vi "Create Test Method Dialog.vi"(11 "Class Ref":refnum<vi>) -> ()   [LabVIEW 2013, in "Scripter.lvlib"]
uses:
  Scripter.lvlib
  _td Dialog Data.ctl
panel:
  out "Methods List":string[](array[string])
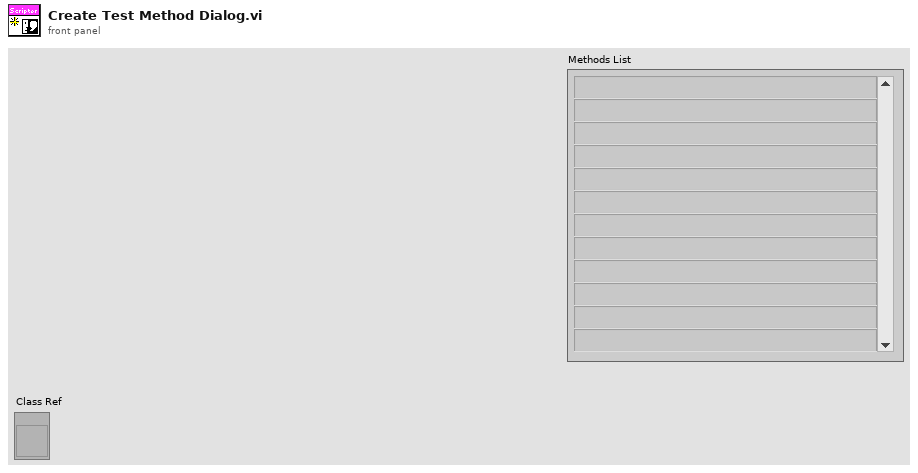
[diagram p1: front panel]
types:
  T1 = enum32{"Invalid", "Standard", "Closed", "Hidden", "Minimized", "Maximized"}
  T2 = enum32{"invalid app kind", "Development System", "Run Time System", "Student Edition", "Embedded LabVIEW", "Evaluation", "Custom"}
  T3 = typedef "Scripter.lvlib/_td Dialog Data.ctl" = cluster{"Core":cluster{"Current VI Reference":refnum<vi>, "Close Panel on Exit?":bool}, "Class Ref":refnum<vi>, "Class Folder Path":path, "Method Name":string, "Methods List":string[], "Templates Folder Path":path, "Template VIs":path[], "Template VIs List":string[], "Use Template?":bool}
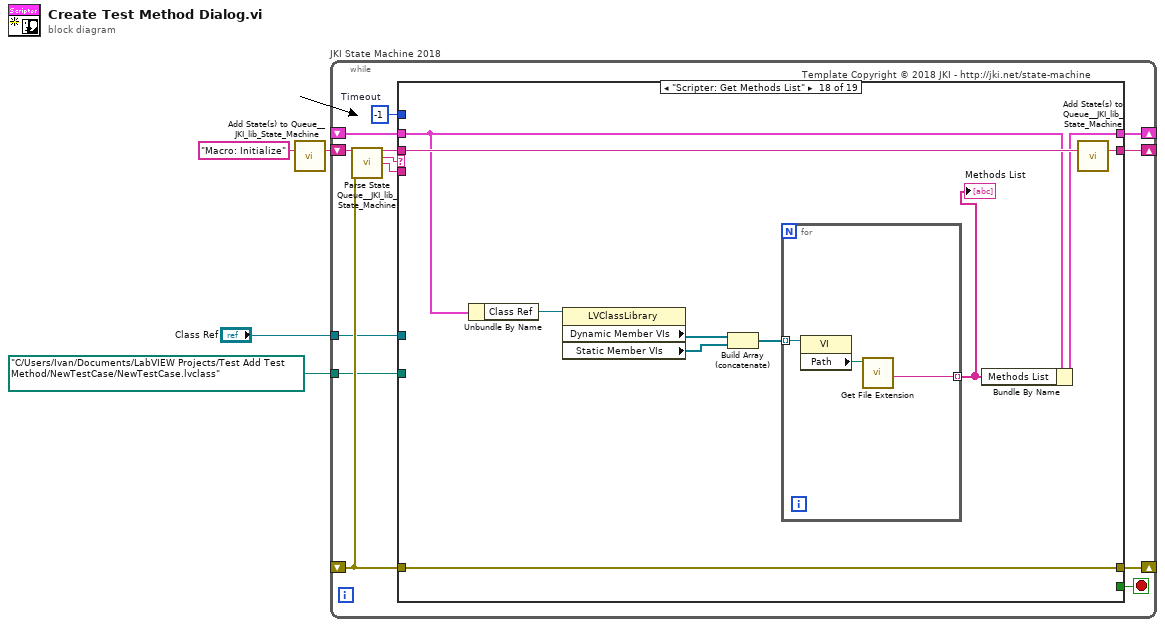
[diagram p0: block diagram]
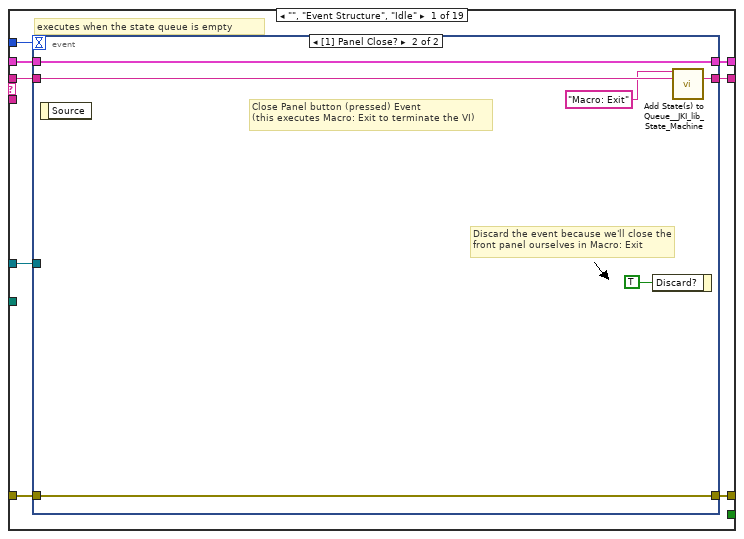
[diagram p2: hidden frame]
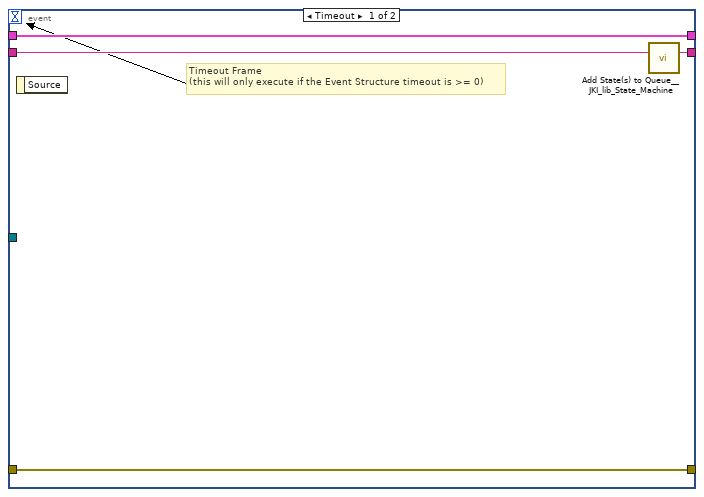
[diagram p3: hidden frame]
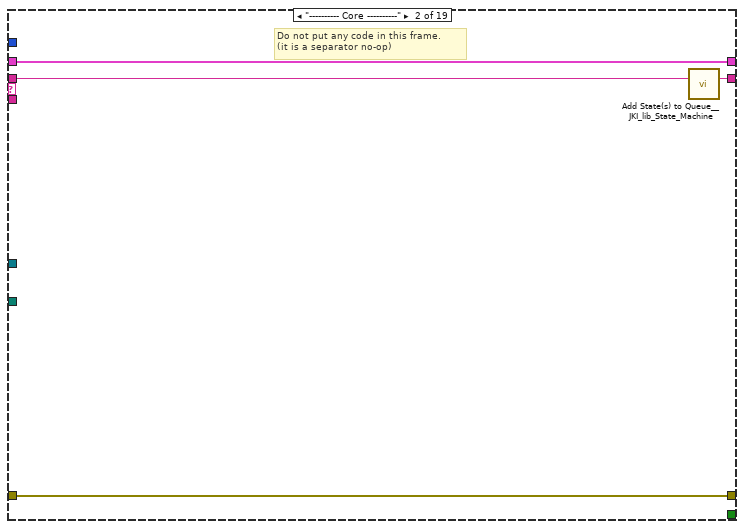
[diagram p4: hidden frame]
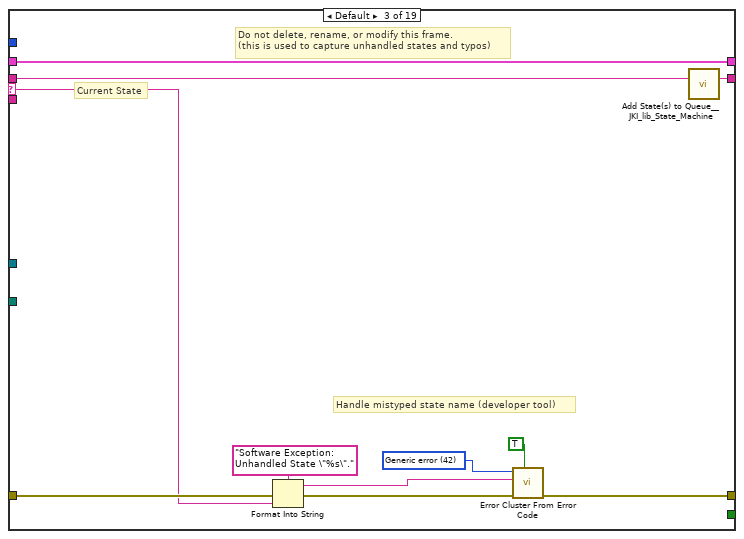
[diagram p5: hidden frame]
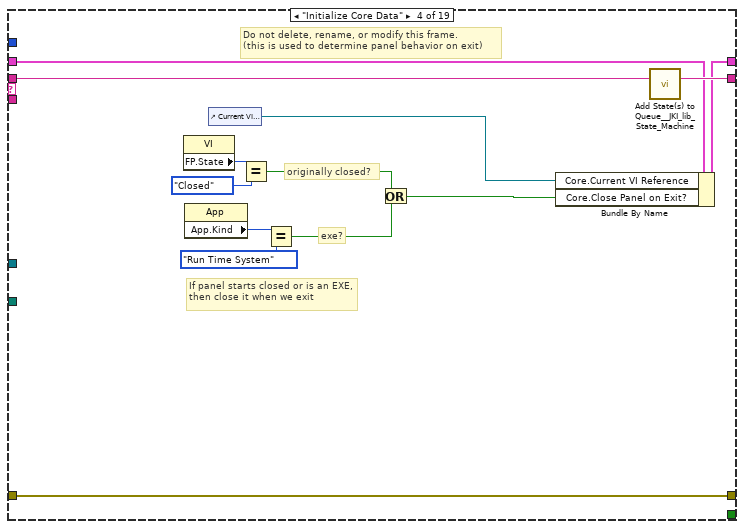
[diagram p6: hidden frame]
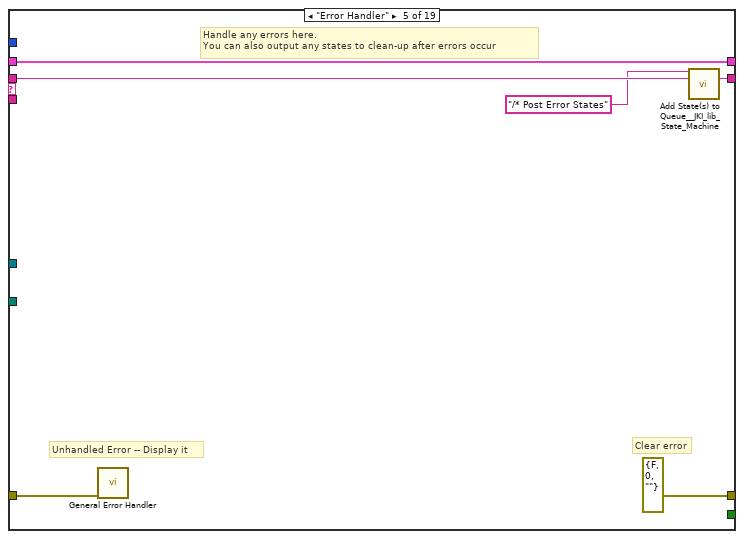
[diagram p7: hidden frame]
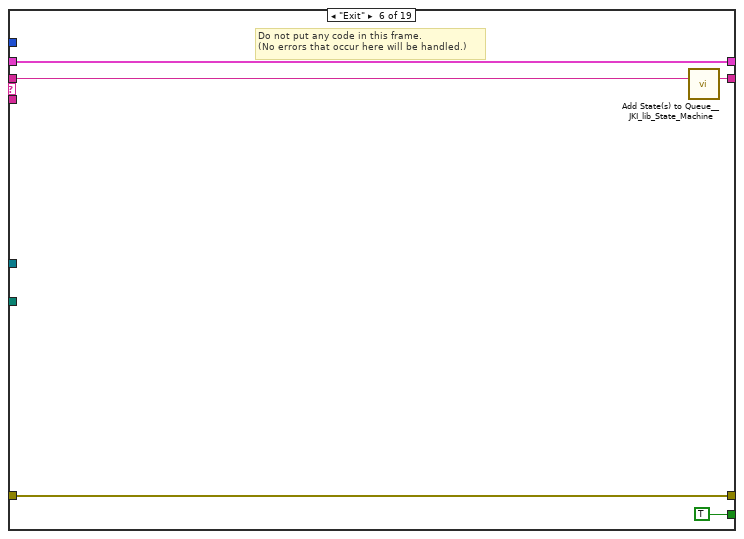
[diagram p8: hidden frame]
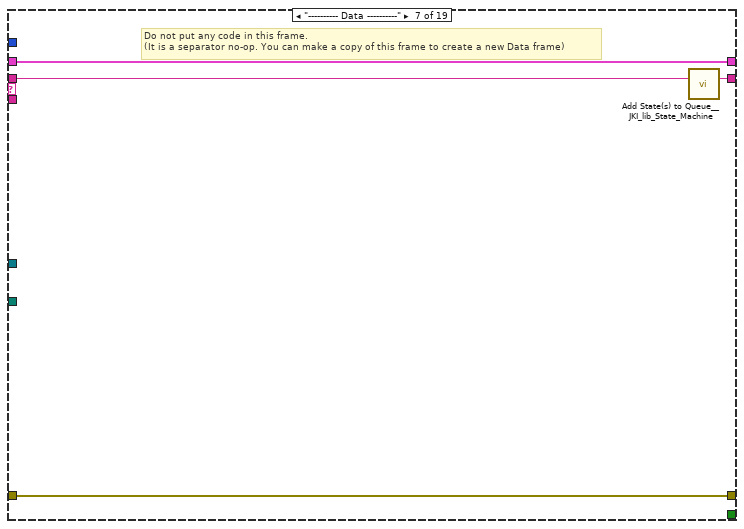
[diagram p9: hidden frame]
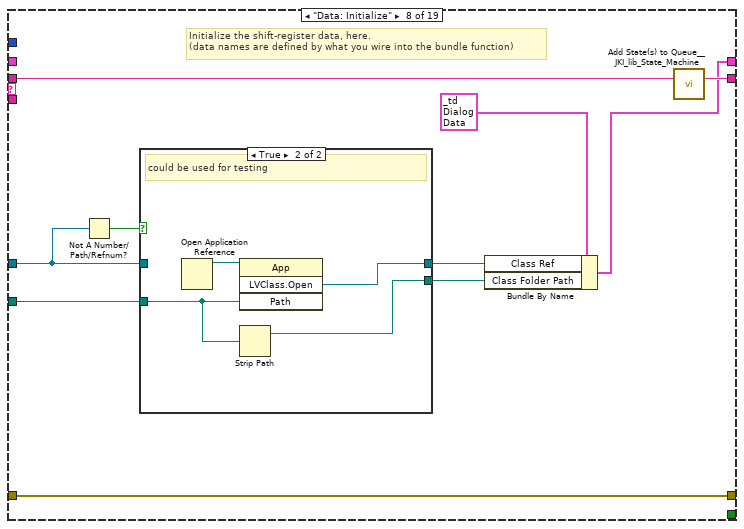
[diagram p10: hidden frame]
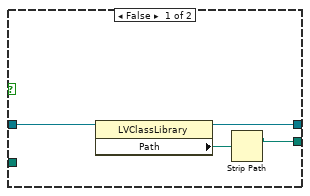
[diagram p11: hidden frame]
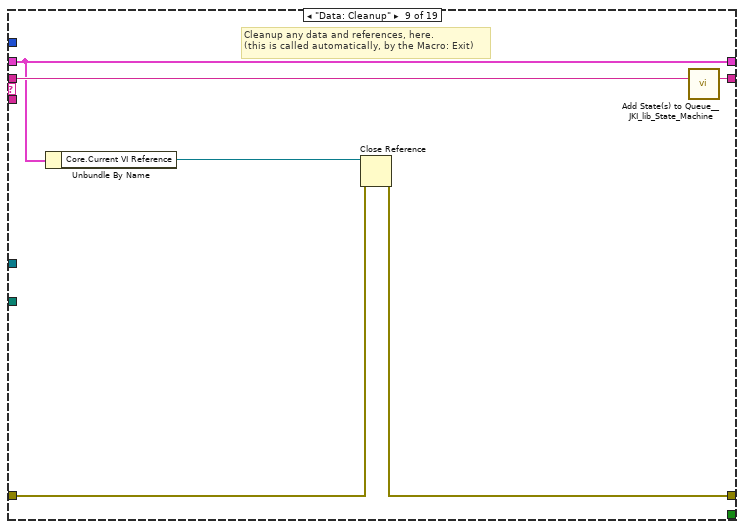
[diagram p12: hidden frame]
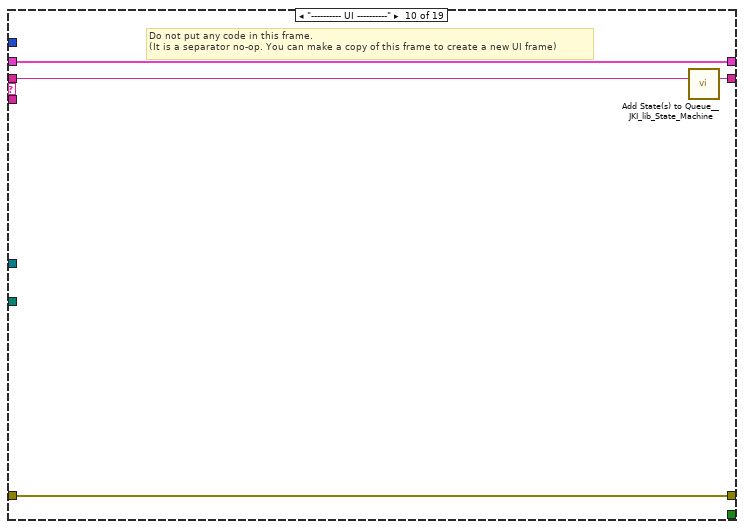
[diagram p13: hidden frame]
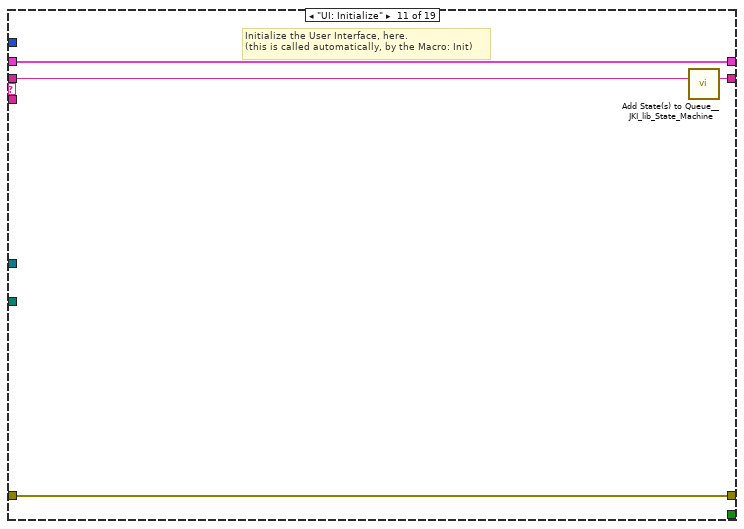
[diagram p14: hidden frame]
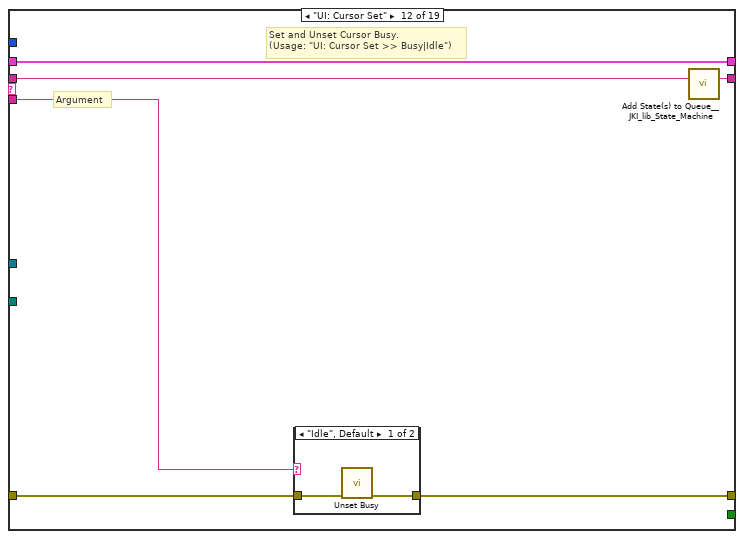
[diagram p15: hidden frame]
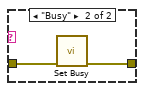
[diagram p16: hidden frame]
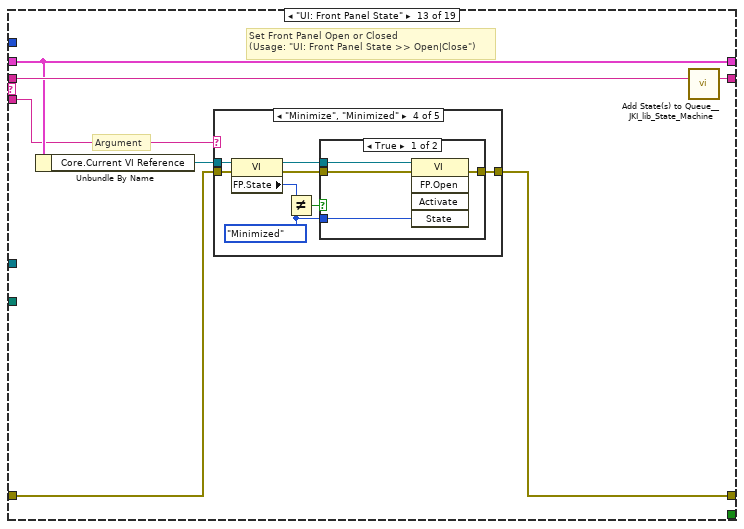
[diagram p17: hidden frame]
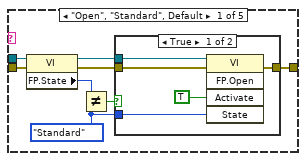
[diagram p18: hidden frame]
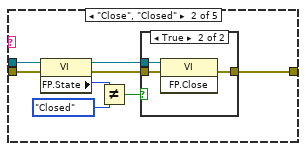
[diagram p20: hidden frame]
diagram:
  n1 = call <vilib>:"Add State(s) to Queue__JKI_lib_State_Machine.vi"("State(s) in (\"\")"="Macro: Initialize") -> ("States Out"=w4:string)  [unwired: 14 in]
  n2 = while "JKI State Machine 2018" {
    shift-right: [w10] -> _
    shift-left: _ -> [w9]
    shift-right: [w13] -> _
    shift-left: _ -> [w7]
    shift-right: [w12] -> _
    shift-left: w4 -> [w14]
    tunnel: "Class Ref" -> [w6]
    tunnel: path "C:/Users/Ivan/Documents/LabVIEW Projects/Test Add Test Method/NewTestCase/NewTestCase.lvclass" -> [w5]
    stop <- w11 stop-if-true
    w8 = -1  # Timeout
    # "Template Copyright © 2018 JKI - http://jki.net/state-machine"
    n3 = call <vilib>:"Parse State Queue__JKI_lib_State_Machine.vi"("State Queue"=w14, "Error In (no error)"=w7) -> ("Remaining States"=w16:string, "Current State"=w17:string, "Arguments"=w15:string)  [unwired: 11 in]
    n4 = case shown="\"Scripter: Get Methods List\"" w17 {
      selector: w17 -> [_ _ w40 _ _ _ _ _ _ _ _ _ _ _ _ _ _ _ _]
      tunnel: w16 -> [w25 w39 w44 w63 w69 w74 w78 w88 w102 w106 w110 w116 w127 w196 w201 w211 w215 w225 w232]
      tunnel: w15 -> [_ _ _ _ _ _ _ _ _ _ _ w111 w121 _ _ _ _ _ _]
      tunnel: w9 -> [w23 w36 w42 w56 w66 w72 w75 _ w97 w103 w108 w114 w123 w193 w198 w208 w212 w222 w229]
      tunnel: [w22 w37 w46 w60 errorcluster {"status"=FALSE, "code"=0, "source"=""} ("error out") w71 w76 w86 w98 w104 w107 w112 w124 w194 w199 w209 w213 w223 w230] -> w13
      tunnel: w7 -> [w21 w37 w45 w60 w65 w71 w76 w86 w99 w104 w107 w113 w125 w194 w199 w209 w213 w223 w230]
      tunnel: [w24 w38 w43 w62 w68 w73 w77 w87 w101 w105 w109 w115 w126 w195 w200 w210 w214 w224 w231] -> w12
      tunnel: [_ _ _ _ _ TRUE _ _ _ _ _ _ _ _ _ _ _ _ _] -> w11
      tunnel: [w20 w36 w42 w61 w66 w72 w75 w84 w97 w103 w108 w114 w123 w193 w198 w208 w212 w217 w229] -> w10
      tunnel: w8 -> [w19 _ _ _ _ _ _ _ _ _ _ _ _ _ _ _ _ _ _]
      tunnel: w6 -> [w18 _ _ _ _ _ _ w82 _ _ _ _ _ _ _ _ _ _ _]
      tunnel: w5 -> [_ _ _ _ _ _ _ w80 _ _ _ _ _ _ _ _ _ _ _]
      frame "", "Event Structure", "Idle" {
        # "executes when the state queue is empty"
        n5 = event shown="[1] Panel Close?" {
          selector: _ -> [_ _]
          dyn-events: _ -> [_ _]
          timeout: w19 -> [_ _]
          tunnel: w25 -> [w29 w35]
          tunnel: [w28 w34] -> w24
          tunnel: w23 -> [w26 w32]
          tunnel: [w27 w33] -> w22
          tunnel: w21 -> [w27 w33]
          tunnel: [w26 w32] -> w20
          tunnel: w18 -> [_ _]
          event Timeout {
            # "Timeout Frame\n(this will only execute if the Event Structure timeout is >= 0)"
            n6 = event-data() -> ()  [unwired: 1 in, 1 out]
            n7 = call <vilib>:"Add State(s) to Queue__JKI_lib_State_Machine.vi"("State(s) in (\"\")"=w29) -> ("States Out"=w28:string)  [unwired: 14 in]
          }
          event Panel Close? {
            # "Discard the event because we'll close the front panel ourselves in Macro: Exit"
            # "Close Panel button (pressed) Event\n(this executes Macro: Exit to terminate the VI)"
            n8 = event-data() -> ()  [unwired: 1 in, 1 out]
            n9 = event-data("Discard?"=TRUE) -> ()  [unwired: 1 in, 1 out]
            n10 = call <vilib>:"Add State(s) to Queue__JKI_lib_State_Machine.vi"("State(s) in Front (\"\")"="Macro: Exit", "State(s) in (\"\")"=w35) -> ("States Out"=w34:string)  [unwired: 13 in]
          }
        }
      }
      frame "---------- Core ----------" {
        # "Do not put any code in this frame.\n(it is a separator no-op)"
        n11 = call <vilib>:"Add State(s) to Queue__JKI_lib_State_Machine.vi"("State(s) in (\"\")"=w39) -> ("States Out"=w38:string)  [unwired: 14 in]
      }
      frame Default {
        w49 = 42 items=["No error", "Argument error", "Memory is full", "Out of zone", "End of file", "File already open", "Generic file I/O error", "File not found", "File permission error", "Disk is full", "Duplicate path", "Too many files open", "System feature not enabled", "Resource file not found", "Cannot add resource", "Resource not found", "Image not found", "Image memory error", "Pen does not exist", "Config type invalid", "Config token not found", "Config parse error", "Config memory error", "Bad external code format", "Bad external code offset", "External code not present", "Null window", "Destroy window error", "Null menu", "Print aborted", "Bad print record", "Print driver error", "Windows error during printing", "Memory error during printing", "Print dialog error", "Generic print error", "Invalid device refnum", "Device not found", "Device parameter error", "Device unit error", "Cannot open device", "Device call aborted", "Generic error", "Cancelled by user", "Object ID too low", "Object ID too high", "Object not in heap", "Unknown heap", "Unknown object (invalid DefProc)", "Unknown object (DefProc not in table)", "Message out of range", "Invalid (null) method", "Unknown message", "Manager call not supported", "Bad address", "Network operation in progress", "Network operation timed out", "Connection is busy", "Network attribute not supported", "Network error", "Address in use", "System out of memory", "Connection aborted", "Connection refused", "Not connected", "Already connected", "Connection closed", "Initialization error (interapplication manager)", "Bad occurrence", "Wait on unbound occurrence handler", "Occurrence queue overflow", "Datalog type conflict", "Unused", "Unrecognized type (interapplication manager)", "Memory corrupt", "Failed to make temporary DLL", "Old CIN version", "Drag socket not found", "Failed to load drop-object", "Failed to register OLE object", "Failed to release OLE object", "Format specifier type mismatch", "Unknown format specifier", "Too few format specifiers", "Too many format specifiers", "Scan failed", "Newer CIN version", "Error converting to variant", "Runtime menu error", "Password tampered", "Variant attribute not found", "Incompatible variant data type", "Event data is not available", "Event Store is not present", "Occurrence is not found", "Event Queue is not created", "Event info is not available", "Refnum passed is NULL", "Error retrieving Class GUID", "Error retrieving CoClass GUID", "Error retrieving TypeLib GUID.", "Bad built application magic bytes.", "Specific driver is different from the specific driver associated with the Logical Name.", "There is no session opened to the class driver.", "Max Error", "MAX - Error with config objects", "MAX - Error loading configuration", "MAX - Group not supported"]
        # "Current State"
        # "Do not delete, rename, or modify this frame.\n(this is used to capture unhandled states and typos)"
        # "Handle mistyped state name (developer tool)"
        n12 = Format Into String(format string="Software Exception: Unhandled State \"%s\"." ("message"), error in=w45, w40) -> (resulting string=w48:string, error out=w47:errorcluster)  [unwired: 1 in]
        n13 = call <vilib>:"Error Cluster From Error Code.vi"("show call chain? (False)"=TRUE, "error in (no error)"=w47, "error message (\"\")"=w48, "error code (0)"=w49) -> ("error out"=w46:errorcluster)  [unwired: 5 in]
        n14 = call <vilib>:"Add State(s) to Queue__JKI_lib_State_Machine.vi"("State(s) in (\"\")"=w44) -> ("States Out"=w43:string)  [unwired: 14 in]
      }
      frame "Initialize Core Data" {
        # "Do not delete, rename, or modify this frame.\n(this is used to determine panel behavior on exit)"
        # "originally closed?"
        # "exe?"
        # "If panel starts closed or is an EXE, then close it when we exit"
        n15 = property class="VI"() -> ("FP.State"=w53:T1)  [unwired: 2 in, 2 out]
        n16 = property class="App"() -> ("App.Kind"=w59:T2)  [unwired: 2 in, 2 out]
        n17 = control-ref of="Current VI Reference"() -> (w54:refnum<vi>)
        n18 = Equal?(x=w53, y=T1."Closed" ("Front Panel Window:State")) -> (x = y?=w51:bool)
        n19 = Equal?(x=w59, y=T2."Run Time System" ("Application:Kind")) -> (x = y?=w57:bool)
        n20 = Or(x=w51, y=w57) -> (x .or. y?=w55:bool)
        n21 = Bundle By Name(cluster=w56, "Core.Current VI Reference"=w54, "Core.Close Panel on Exit?"=w55) -> (w61:T3)
        n22 = call <vilib>:"Add State(s) to Queue__JKI_lib_State_Machine.vi"("State(s) in (\"\")"=w63) -> ("States Out"=w62:string)  [unwired: 14 in]
      }
      frame "Error Handler" {
        # "Unhandled Error -- Display it"
        # "Handle any errors here.\nYou can also output any states to clean-up after errors occur"
        # "Clear error"
        n23 = call <vilib>:"General Error Handler.vi"("error in (no error)"=w65) -> ()  [unwired: 10 in, 5 out]
        n24 = call <vilib>:"Add State(s) to Queue__JKI_lib_State_Machine.vi"("State(s) in Front (\"\")"="/* Post Error States", "State(s) in (\"\")"=w69) -> ("States Out"=w68:string)  [unwired: 13 in]
      }
      frame "Exit" {
        # "Do not put any code in this frame.\n(No errors that occur here will be handled.)"
        n25 = call <vilib>:"Add State(s) to Queue__JKI_lib_State_Machine.vi"("State(s) in (\"\")"=w74) -> ("States Out"=w73:string)  [unwired: 14 in]
      }
      frame "---------- Data ----------" {
        # "Do not put any code in this frame.\n(It is a separator no-op. You can make a copy of this frame to create a new Data frame)"
        n26 = call <vilib>:"Add State(s) to Queue__JKI_lib_State_Machine.vi"("State(s) in (\"\")"=w78) -> ("States Out"=w77:string)  [unwired: 14 in]
      }
      frame "Data: Initialize" {
        # "Initialize the shift-register data, here.\n(data names are defined by what you wire into the bundle function)"
        n27 = Not A Number/Path/Refnum?(number/path/refnum=w82) -> (NaN/Path/Refnum?=w83:bool)
        n28 = case shown="True" w83 {
          tunnel: w82 -> [w92 _]
          tunnel: [w91 w95] -> w81
          tunnel: w80 -> [_ w94]
          tunnel: [w89 w93] -> w79
          frame False {
            n29 = property class="LVClassLibrary"(reference=w92) -> (reference out=w91:refnum<vi>, "Path"=w90:path)  [unwired: 1 in, 1 out]
            n30 = Strip Path(path=w90) -> (stripped path=w89:path)  [unwired: 1 out]
          }
          frame True {
            # "could be used for testing"
            n31 = Open Application Reference() -> (3:w96:refnum<vi>)  [unwired: 4 in, 1 out]
            n32 = invoke class="App" method="LVClass.Open"(reference=w96, "Path"=w94) -> ("LVClass.Open"=w95:refnum<vi>)  [unwired: 2 in, 3 out]
            n33 = Strip Path(path=w94) -> (stripped path=w93:path)  [unwired: 1 out]
          }
        }
        n34 = Bundle By Name(cluster=T3 {"Core"={"Current VI Reference"=refnum, "Close Panel on Exit?"=FALSE}, "Class Ref"=refnum, "Class Folder Path"=path "", "Method Name"="", "Methods List"=[], "Templates Folder Path"=path "", "Template VIs"=[], "Template VIs List"=[], "Use Template?"=FALSE} ("Dialog Data"), "Class Ref"=w81, "Class Folder Path"=w79) -> (w84:T3)
        n35 = call <vilib>:"Add State(s) to Queue__JKI_lib_State_Machine.vi"("State(s) in (\"\")"=w88) -> ("States Out"=w87:string)  [unwired: 14 in]
      }
      frame "Data: Cleanup" {
        # "Cleanup any data and references, here.\n(this is called automatically, by the Macro: Exit)"
        n36 = Unbundle By Name(w97) -> ("Core.Current VI Reference"=w100:refnum<vi>)
        n37 = Close Reference(reference=w100, error in (no error)=w99) -> (error out=w98:errorcluster)
        n38 = call <vilib>:"Add State(s) to Queue__JKI_lib_State_Machine.vi"("State(s) in (\"\")"=w102) -> ("States Out"=w101:string)  [unwired: 14 in]
      }
      frame "---------- UI ----------" {
        # "Do not put any code in this frame.\n(It is a separator no-op. You can make a copy of this frame to create a new UI frame)"
        n39 = call <vilib>:"Add State(s) to Queue__JKI_lib_State_Machine.vi"("State(s) in (\"\")"=w106) -> ("States Out"=w105:string)  [unwired: 14 in]
      }
      frame "UI: Initialize" {
        # "Initialize the User Interface, here.\n(this is called automatically, by the Macro: Init)"
        n40 = call <vilib>:"Add State(s) to Queue__JKI_lib_State_Machine.vi"("State(s) in (\"\")"=w110) -> ("States Out"=w109:string)  [unwired: 14 in]
      }
      frame "UI: Cursor Set" {
        # "Argument"
        # "Set and Unset Cursor Busy.\n(Usage: \"UI: Cursor Set >> Busy|Idle\")"
        n41 = case shown="\"Idle\", Default" w111 {
          tunnel: w113 -> [w118 w120]
          tunnel: [w117 w119] -> w112
          frame "Idle", Default {
            n42 = call <vilib>:"Unset Busy.vi"("error in (no error)"=w118) -> ("error out"=w117:errorcluster)  [unwired: 10 in]
          }
          frame "Busy" {
            n43 = call <vilib>:"Set Busy.vi"("error in (no error)"=w120) -> ("error out"=w119:errorcluster)  [unwired: 9 in, 1 out]
          }
        }
        n44 = call <vilib>:"Add State(s) to Queue__JKI_lib_State_Machine.vi"("State(s) in (\"\")"=w116) -> ("States Out"=w115:string)  [unwired: 14 in]
      }
      frame "UI: Front Panel State" {
        # "Argument"
        # "Set Front Panel Open or Closed\n(Usage: \"UI: Front Panel State >> Open|Close\")"
        n45 = Unbundle By Name(w123) -> ("Core.Current VI Reference"=w122:refnum<vi>)
        n46 = case shown="\"Minimize\", \"Minimized\"" w121 {
          tunnel: w125 -> [w133 w148 w159 w172 w185]
          tunnel: [w135 w149 w161 w174 w187] -> w124
          tunnel: w122 -> [w134 w146 w160 w173 w186]
          frame "Open", "Standard", Default {
            w128 = T1."Standard" ("State")
            n47 = property class="VI"(reference=w134, error in=w133) -> (reference out=w131:refnum<vi>, error out=w132:errorcluster, "FP.State"=w130:T1)
            n48 = Not Equal?(x=w130, y=w128) -> (x != y?=w129:bool)
            n49 = case shown="True" w129 {
              tunnel: [w139 w141] -> w135
              tunnel: w132 -> [w138 w141]
              tunnel: w131 -> [w137 _]
              tunnel: w128 -> [w136 _]
              frame True {
                n50 = invoke class="VI" method="FP.Open"(reference=w137, error in=w138, "Activate"=TRUE, "State"=w136) -> (error out=w139:errorcluster)  [unwired: 1 in, 4 out]
              }
              frame False {
              }
            }
          }
          frame "Close", "Closed" {
            n51 = property class="VI"(reference=w146, error in=w148) -> (reference out=w145:refnum<vi>, error out=w147:errorcluster, "FP.State"=w143:T1)
            n52 = Not Equal?(x=w143, y=T1."Closed" ("Front Panel Window:State")) -> (x != y?=w142:bool)
            n53 = case shown="True" w142 {
              tunnel: [w150 w153] -> w149
              tunnel: w147 -> [w150 w152]
              tunnel: w145 -> [_ w151]
              frame False {
              }
              frame True {
                n54 = invoke class="VI" method="FP.Close"(reference=w151, error in=w152) -> (error out=w153:errorcluster)  [unwired: 1 in, 2 out]
              }
            }
          }
          frame "Hidden", "Hide" {
            w154 = T1."Hidden" ("State")
            n55 = property class="VI"(reference=w160, error in=w159) -> (reference out=w157:refnum<vi>, error out=w158:errorcluster, "FP.State"=w156:T1)
            n56 = Not Equal?(x=w156, y=w154) -> (x != y?=w155:bool)
            n57 = case shown="True" w155 {
              tunnel: [w165 w166] -> w161
              tunnel: w158 -> [w164 w166]
              tunnel: w157 -> [w163 _]
              tunnel: w154 -> [w162 _]
              frame True {
                n58 = invoke class="VI" method="FP.Open"(reference=w163, error in=w164, "State"=w162) -> (error out=w165:errorcluster)  [unwired: 2 in, 4 out]
              }
              frame False {
              }
            }
          }
          frame "Minimize", "Minimized" {
            w167 = T1."Minimized" ("State")
            n59 = property class="VI"(reference=w173, error in=w172) -> (reference out=w170:refnum<vi>, error out=w171:errorcluster, "FP.State"=w169:T1)
            n60 = Not Equal?(x=w169, y=w167) -> (x != y?=w168:bool)
            n61 = case shown="True" w168 {
              tunnel: [w178 w179] -> w174
              tunnel: w171 -> [w177 w179]
              tunnel: w170 -> [w176 _]
              tunnel: w167 -> [w175 _]
              frame True {
                n62 = invoke class="VI" method="FP.Open"(reference=w176, error in=w177, "State"=w175) -> (error out=w178:errorcluster)  [unwired: 2 in, 4 out]
              }
              frame False {
              }
            }
          }
          frame "Maximize", "Maximized" {
            w180 = T1."Maximized" ("State")
            n63 = property class="VI"(reference=w186, error in=w185) -> (reference out=w183:refnum<vi>, error out=w184:errorcluster, "FP.State"=w182:T1)
            n64 = Not Equal?(x=w182, y=w180) -> (x != y?=w181:bool)
            n65 = case shown="True" w181 {
              tunnel: [w191 w192] -> w187
              tunnel: w184 -> [w190 w192]
              tunnel: w183 -> [w189 _]
              tunnel: w180 -> [w188 _]
              frame True {
                n66 = invoke class="VI" method="FP.Open"(reference=w189, error in=w190, "State"=w188) -> (error out=w191:errorcluster)  [unwired: 2 in, 4 out]
              }
              frame False {
              }
            }
          }
        }
        n67 = call <vilib>:"Add State(s) to Queue__JKI_lib_State_Machine.vi"("State(s) in (\"\")"=w127) -> ("States Out"=w126:string)  [unwired: 14 in]
      }
      frame "---------- Macro ----------" {
        # "Do not put any code in this frame.\n(It is a separator no-op. You can make a copy of this frame to create a new Macro frame)"
        n68 = call <vilib>:"Add State(s) to Queue__JKI_lib_State_Machine.vi"("State(s) in (\"\")"=w196) -> ("States Out"=w195:string)  [unwired: 14 in]
      }
      frame "Macro: Initialize" {
        w197 = "Data: Initialize\nInitialize Core Data\nUI: Initialize\nUI: Front Panel State >> Open\nScripter: Get Methods List"  # Data: Initialize Initialize Core Data UI: Initialize UI: Front Panel State >> Open Scripter: Get Methods List
        # "Initialization Macro\n(This is called once, when the VI starts)"
        n69 = call <vilib>:"Add State(s) to Queue__JKI_lib_State_Machine.vi"("State(s) in Front (\"\")"=w197, "State(s) in (\"\")"=w201) -> ("States Out"=w200:string)  [unwired: 13 in]
      }
      frame "Macro: Exit" {
        # "Exit Macro\n(This is called once, when the VI exits)"
        n70 = Unbundle By Name(w208) -> ("Core.Close Panel on Exit?"=w207:bool)
        n71 = Select(t="UI: Front Panel State >> Close", s=w207, f="") -> (s? t:f=w204:string)
        n72 = call <vilib>:"Add State(s) to Queue__JKI_lib_State_Machine.vi"("State(s) in (\"\")"=w204, "State(s) at Back (\"\")"="Data: Cleanup\nExit") -> ("States Out"=w202:string)  [unwired: 13 in]
        n73 = call <vilib>:"Add State(s) to Queue__JKI_lib_State_Machine.vi"("State(s) in Front (\"\")"=w202, "State(s) in (\"\")"=w211) -> ("States Out"=w210:string)  [unwired: 13 in]
      }
      frame "---------- Scripter ----------" {
        # "Template Separator\n(You can make a copy of, or modify, this frame)"
        n74 = call <vilib>:"Add State(s) to Queue__JKI_lib_State_Machine.vi"("State(s) in (\"\")"=w215) -> ("States Out"=w214:string)  [unwired: 14 in]
      }
      frame "Scripter: Get Methods List" {
        n75 = Unbundle By Name(w222) -> ("Class Ref"=w221:refnum<vi>)
        n76 = property class="LVClassLibrary"(reference=w221) -> ("Dynamic Member VIs"=w220:refnum<vi>[], "Static Member VIs"=w219:refnum<vi>[])  [unwired: 1 in, 2 out]
        n77 = Build Array (concatenate)(w220, w219) -> (w218:refnum<vi>[])
        n78 = for {
          tunnel: w218 -> [w228] mode=indexing
          tunnel: [w226] -> w216 mode=indexing
          n79 = property class="VI"(reference=w228) -> ("Path"=w227:path)  [unwired: 1 in, 2 out]
          n80 = call <vilib>:"Get File Extension.vi"("file"=w227) -> ("filename without extension"=w226:string)  [unwired: 7 in, 3 out]
        }
        "Methods List" <- w216
        n81 = Bundle By Name(cluster=w222, "Methods List"=w216) -> (w217:T3)
        n82 = call <vilib>:"Add State(s) to Queue__JKI_lib_State_Machine.vi"("State(s) in (\"\")"=w225) -> ("States Out"=w224:string)  [unwired: 14 in]
      }
      frame "Scripter: 2" {
        # "Your code here.\n(You can make a copy of, or modify, this frame)"
        n83 = call <vilib>:"Add State(s) to Queue__JKI_lib_State_Machine.vi"("State(s) in (\"\")"=w232) -> ("States Out"=w231:string)  [unwired: 14 in]
      }
    }
  }
